vi "DAQ_OPC UA.vi"() -> (0 "Error Out":errorcluster)   [LabVIEW 2017]
uses:
  <vilib>/dex/Flush And Wait Empty Condition.ctl
  <vilib>/Platform/TimedLoop/XDataNode/timing_clust.ctl
  <vilib>/Platform/TimedLoop/XDataNode/nitl_modes.ctl
  <vilib>/Platform/TimedLoop/XDataNode/wakeup.ctl
  <vilib>/DAQmx/read.llb/DAQmx Read (Analog 1D DBL NChan 1Samp).vi
  <vilib>/DAQmx/miscellaneous.llb/DAQmx Fill In Error Info.vi
  <vilib>/Platform/TimedLoop/XDataNode/XDataNode.xnode
  <vilib>/Platform/TimedLoop/XDataNode/XDNodeRunTimeDep.lvlib
  <resource>/objmgr/ni.dex.rc
panel:
  out "Producer Loop Time":i64
  out "Consumer Loop Time":u32
  out "Time":dbl
  out "Available Elements for Writing":i32
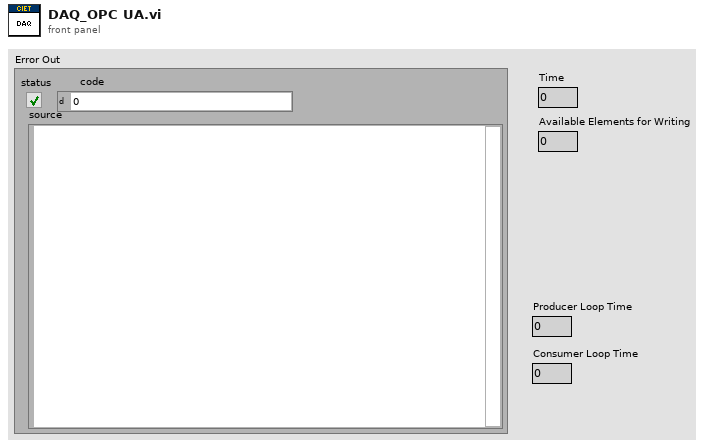
[diagram p1: front panel]
types:
  T1 = typedef "Flush And Wait Empty Condition.ctl" = u8
  T2 = typedef "XDNodeRunTimeDep.lvlib/timing_clust.ctl" = cluster{"Expected End [f-1]":u64, "Actual End [f-1]":u64, "Finished Late? [f-1]":bool, "Expected End [i-1]":u64, "Actual End [i-1]":u64, "Finished Late? [i-1]":bool, "Expected Start [i]":u64, "Actual Start [i]":u64, "Expected Start [f]":u64, "Actual Start [f]":u64, "Source Name":string, "Structure Name":string, "Period":i64, "Deadline":i64, "Offset":i64, "Start":i64, "Priority":i32, "Timeout":i32, "Mode":T3, "Wakeup Reason":T4, "Error":errorcluster, "Source Type":string, "Secondary Source Type":string, "Global End Time":u64, "Global Start Time":u64, "Frame Duration":u64, "Iteration Duration":u64, "Assigned CPU":i32, "I/O Scan Engine Mode":u32}
  T3 = typedef "XDNodeRunTimeDep.lvlib/nitl_modes.ctl" = enum32{"No Change", "Process missed periods, maintain original phase", "Discard missed periods, maintain original phase", "Process missed periods, ignore original phase", "Discard missed periods, ignore original phase"}
  T4 = typedef "XDNodeRunTimeDep.lvlib/wakeup.ctl" = enum32{"Normal", "Aborted", "Asynchronous wakeup", "Timing source error", "Timed loop error", "Timeout"}
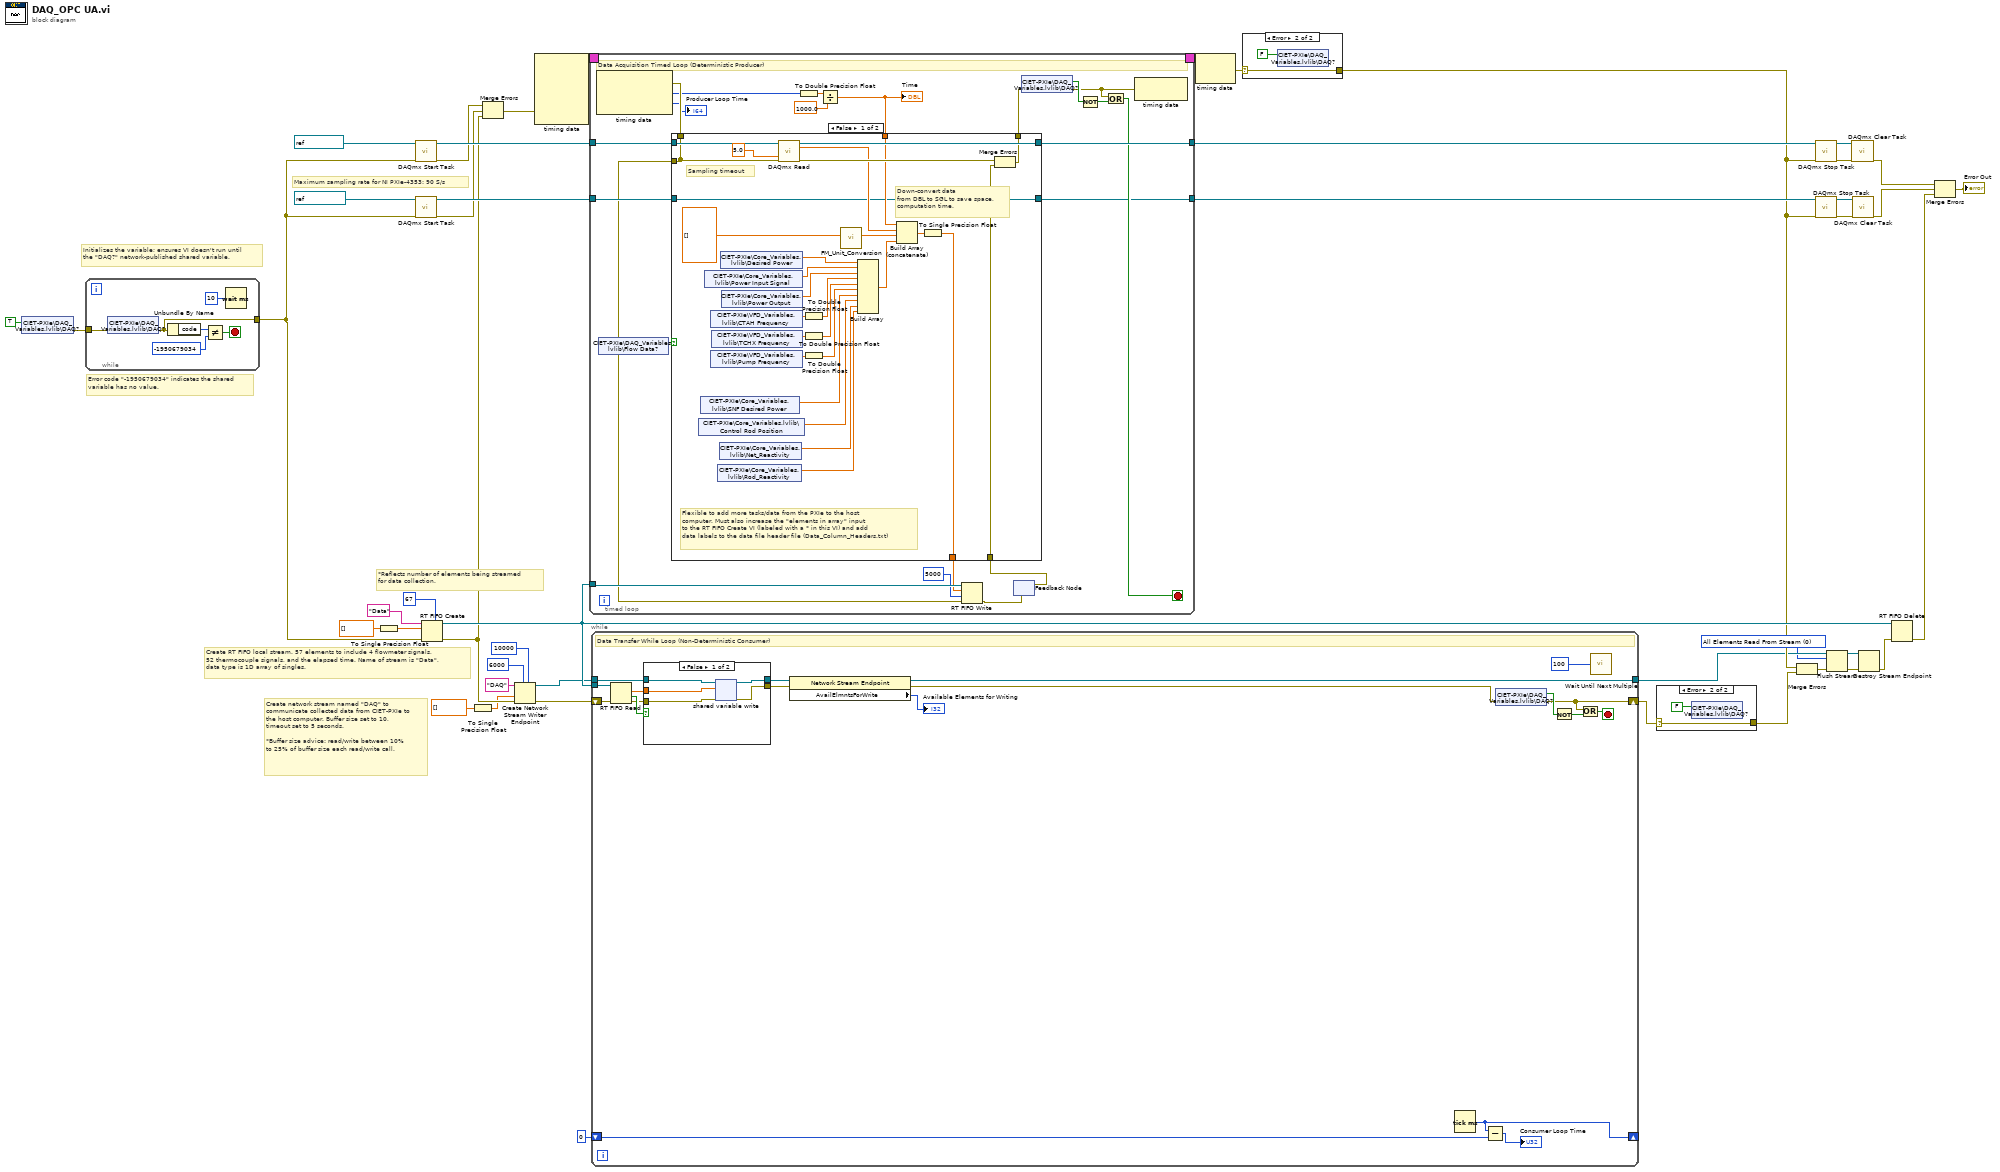
[diagram p0: block diagram]
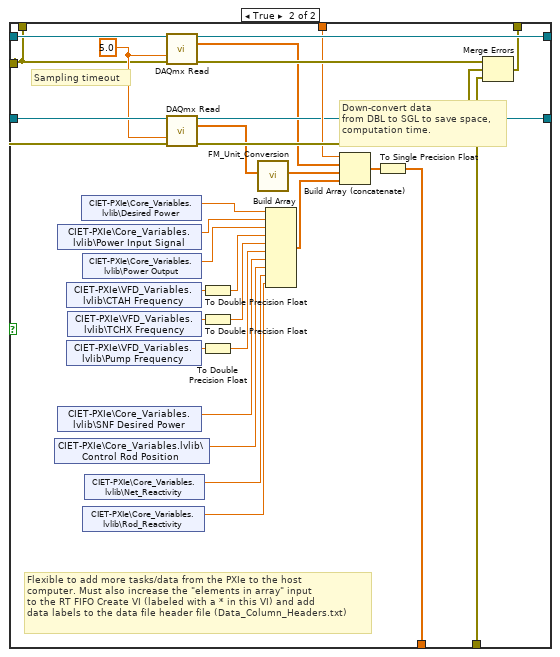
[diagram p5: hidden frame]
diagram:
  w2 = T1 0 items=["All Elements Read From Stream", "All Elements Available for Reading"] ("wait condition")
  # "*Reflects number of elements being streamed\nfor data collection."
  # "Create RT FIFO local stream. 57 elements to include 4 flowmeter signals,\n52 thermocouple signals, and the elapsed time. Name of stream is \"Data\",\ndata type is 1D array of singles."
  # "Create network stream named \"DAQ\" to communicate collected data from CIET-PXIe to the host computer. Buffer size set to 10, timeout set to 5 seconds. \n\n*Buffer size advice: read/write between 10%\nto 25% of buffer size each read/write call."
  # "Maximum sampling rate for NI PXIe-4353: 90 S/s"
  # "Initializes the variable; ensures VI doesn't run until\nthe \"DAQ?\" network-published shared variable."
  # "Error code \"-1950679034\" indicates the shared\nvariable has no value."
  n1 = shared-variable "CIET-PXIe\\DAQ_Variables.lvlib\\DAQ?"(TRUE ("Active?")) -> (error out=w22:errorcluster)  [unwired: 1 in]
  n2 = while {
    tunnel: w22 -> [w51]
    tunnel: [w50] -> w21
    stop <- w47 stop-if-true
    n3 = shared-variable "CIET-PXIe\\DAQ_Variables.lvlib\\DAQ?"(error in=w51) -> (error out=w50:errorcluster)  [unwired: 1 out]
    n4 = Unbundle By Name(w50) -> ("code"=w49:i32)
    n5 = Not Equal?(x=w49, y=-1950679034) -> (x != y?=w47:bool)
    n6 = Wait (ms)(milliseconds to wait=u32 10) -> ()  [unwired: 1 out]
  }
  n7 = To Single Precision Float(number=dbl[] []) -> (single precision float=w32:sgl[])
  n8 = call <vilib>:"DAQmx Start Task.vi"("task/channels in"=refnum<k21> "CIET-TC", "error in"=w21) -> ("task out"=w42:refnum<k21>, "error out"=w26:errorcluster)  [unwired: 12 in]
  n9 = call <vilib>:"DAQmx Start Task.vi"("task/channels in"=refnum<k21> "CIET-FM", "error in"=w21) -> ("task out"=w41:refnum<k21>, "error out"=w27:errorcluster)  [unwired: 12 in]
  n10 = RT FIFO Create(0:"Data" ("name (unnamed)"), 1:w32, 3:w21, 6:u32 67 ("elements in array (1)")) -> (8:w25:refnum<k33>, 11:w17:errorcluster)  [unwired: 4 in, 1 out]
  n11 = To Single Precision Float(number=dbl[] []) -> (single precision float=w7:sgl[])
  n12 = Merge Errors(w26, w27, w17) -> (w28:errorcluster)
  n13 = Create Network Stream Writer Endpoint(5:10000 ("timeout in ms (-1)"), 7:6000 ("writer buffer size"), 8:w17, 9:w7, 11:"DAQ" ("writer name")) -> (0:w18:errorcluster, 3:w16:refnum<k21>)  [unwired: 2 in]
  n14 = node-c288(w28) -> (w46:T2)  [unwired: 4 in]
  n15 = timed-loop {
    timing: w46 -> [_]
    timing-out: [_] -> w45
    tunnel: w25 -> [w71]
    tunnel: w42 -> [w74]
    tunnel: [w72] -> w36
    tunnel: w41 -> [w73]
    tunnel: [w59] -> w35
    stop <- w66 stop-if-true
    # "Data Acquisition Timed Loop (Deterministic Producer)"
    n16 = node-c288() -> (w69:errorcluster, w60:i64, →"Producer Loop Time":i64)  [unwired: 1 in]
    n17 = shared-variable "CIET-PXIe\\DAQ_Variables.lvlib\\Flow Data?"() -> (w54:bool)  [unwired: 1 in, 1 out]
    n18 = To Double Precision Float(number=w60) -> (double precision float=w63:dbl)
    n19 = Divide(x=w63, y=1000.0) -> (x/y=w62:dbl)
    "Time" <- w62
    n20 = feedback #1() -> (w55:errorcluster)  [unwired: 1 in]
    n21 = case shown="False" w54 {
      tunnel: w74 -> [w102 w132]
      tunnel: w73 -> [w82 w131]
      tunnel: [w100 w129] -> w72
      tunnel: [w98 w127] -> w57
      tunnel: w69 -> [w79 w107]
      tunnel: w55 -> [w80 w124]
      tunnel: [w96 w123] -> w65
      tunnel: w62 -> [w95 w122]
      tunnel: [w82 w121] -> w59
      tunnel: [w79 w107] -> w53
      frame False {
        # "Flexible to add more tasks/data from the PXIe to the host \ncomputer. Must also increase the \"elements in array\" input \nto the RT FIFO Create VI (labeled with a * in this VI) and add\ndata labels to the data file header file (Data_Column_Headers.txt)"
        # "Down-convert data\nfrom DBL to SGL to save space,\ncomputation time."
        # "Sampling timeout"
        n22 = shared-variable "CIET-PXIe\\Core_Variables.lvlib\\Control Rod Position"() -> (w77:dbl)  [unwired: 1 in, 1 out]
        n23 = shared-variable "CIET-PXIe\\Core_Variables.lvlib\\SNF Desired Power"() -> (w78:dbl)  [unwired: 1 in, 1 out]
        n24 = shared-variable "CIET-PXIe\\Core_Variables.lvlib\\Power Input Signal"() -> (w85:dbl)  [unwired: 1 in, 1 out]
        n25 = shared-variable "CIET-PXIe\\VFD_Variables.lvlib\\CTAH Frequency"() -> (w87:sgl)  [unwired: 1 in, 1 out]
        n26 = shared-variable "CIET-PXIe\\VFD_Variables.lvlib\\Pump Frequency"() -> (w89:sgl)  [unwired: 1 in, 1 out]
        n27 = shared-variable "CIET-PXIe\\VFD_Variables.lvlib\\TCHX Frequency"() -> (w88:sgl)  [unwired: 1 in, 1 out]
        n28 = shared-variable "CIET-PXIe\\Core_Variables.lvlib\\Rod_Reactivity"() -> (w75:dbl)  [unwired: 1 in, 1 out]
        n29 = shared-variable "CIET-PXIe\\Core_Variables.lvlib\\Net_Reactivity"() -> (w76:dbl)  [unwired: 1 in, 1 out]
        n30 = shared-variable "CIET-PXIe\\Core_Variables.lvlib\\Desired Power"() -> (w84:dbl)  [unwired: 1 in, 1 out]
        n31 = shared-variable "CIET-PXIe\\Core_Variables.lvlib\\Power Output"() -> (w86:dbl)  [unwired: 1 in, 1 out]
        n32 = call-poly <vilib>:"DAQmx Read.vi"("task/channels in"=w102, "timeout"=5.0, "error in"=w79) -> ("task out"=w100:refnum<k21>, "data"=w94:dbl[], "error out"=w97:errorcluster)  [unwired: 10 in]
        n33 = To Double Precision Float(number=w87) -> (double precision float=w90:dbl)
        n34 = To Double Precision Float(number=w88) -> (double precision float=w91:dbl)
        n35 = To Double Precision Float(number=w89) -> (double precision float=w92:dbl)
        n36 = call "FM_Unit_Conversion.vi"("Input Array [A]"=dbl[] []) -> ("Output Array [kg/h]"=w93:dbl[])  [unwired: 10 in]
        n37 = Build Array(w84, w85, w86, w90, w91, w92, w78, w77, w76, w75) -> (w83:dbl[])
        n38 = Build Array (concatenate)(w95, w94, w93, w83) -> (w99:dbl[])
        n39 = To Single Precision Float(number=w99) -> (single precision float=w98:sgl[])
        n40 = Merge Errors(w97, w80) -> (w96:errorcluster)
      }
      frame True {
        w130 = 5.0 ("timeout")
        # "Flexible to add more tasks/data from the PXIe to the host \ncomputer. Must also increase the \"elements in array\" input \nto the RT FIFO Create VI (labeled with a * in this VI) and add\ndata labels to the data file header file (Data_Column_Headers.txt)"
        # "Down-convert data\nfrom DBL to SGL to save space,\ncomputation time."
        # "Sampling timeout"
        n41 = shared-variable "CIET-PXIe\\Core_Variables.lvlib\\Control Rod Position"() -> (w105:dbl)  [unwired: 1 in, 1 out]
        n42 = shared-variable "CIET-PXIe\\Core_Variables.lvlib\\Power Input Signal"() -> (w110:dbl)  [unwired: 1 in, 1 out]
        n43 = shared-variable "CIET-PXIe\\Core_Variables.lvlib\\SNF Desired Power"() -> (w106:dbl)  [unwired: 1 in, 1 out]
        n44 = shared-variable "CIET-PXIe\\VFD_Variables.lvlib\\CTAH Frequency"() -> (w112:sgl)  [unwired: 1 in, 1 out]
        n45 = shared-variable "CIET-PXIe\\VFD_Variables.lvlib\\Pump Frequency"() -> (w114:sgl)  [unwired: 1 in, 1 out]
        n46 = shared-variable "CIET-PXIe\\VFD_Variables.lvlib\\TCHX Frequency"() -> (w113:sgl)  [unwired: 1 in, 1 out]
        n47 = shared-variable "CIET-PXIe\\Core_Variables.lvlib\\Desired Power"() -> (w109:dbl)  [unwired: 1 in, 1 out]
        n48 = shared-variable "CIET-PXIe\\Core_Variables.lvlib\\Power Output"() -> (w111:dbl)  [unwired: 1 in, 1 out]
        n49 = shared-variable "CIET-PXIe\\Core_Variables.lvlib\\Rod_Reactivity"() -> (w103:dbl)  [unwired: 1 in, 1 out]
        n50 = shared-variable "CIET-PXIe\\Core_Variables.lvlib\\Net_Reactivity"() -> (w104:dbl)  [unwired: 1 in, 1 out]
        n51 = call-poly <vilib>:"DAQmx Read.vi"("task/channels in"=w132, "timeout"=w130, "error in"=w107) -> ("task out"=w129:refnum<k21>, "data"=w120:dbl[], "error out"=w125:errorcluster)  [unwired: 10 in]
        n52 = call-poly <vilib>:"DAQmx Read.vi"("task/channels in"=w131, "timeout"=w130, "error in"=w107) -> ("task out"=w121:refnum<k21>, "data"=w118:dbl[], "error out"=w126:errorcluster)  [unwired: 10 in]
        n53 = To Double Precision Float(number=w112) -> (double precision float=w115:dbl)
        n54 = To Double Precision Float(number=w113) -> (double precision float=w116:dbl)
        n55 = To Double Precision Float(number=w114) -> (double precision float=w117:dbl)
        n56 = call "FM_Unit_Conversion.vi"("Input Array [A]"=w118) -> ("Output Array [kg/h]"=w119:dbl[])  [unwired: 10 in]
        n57 = Build Array(w109, w110, w111, w115, w116, w117, w106, w105, w104, w103) -> (w108:dbl[])
        n58 = Build Array (concatenate)(w122, w120, w119, w108) -> (w128:dbl[])
        n59 = To Single Precision Float(number=w128) -> (single precision float=w127:sgl[])
        n60 = Merge Errors(w125, w126, w124) -> (w123:errorcluster)
      }
    }
    n61 = RT FIFO Write(0:w71, 1:w57, 2:5000 ("timeout in ms (0)"), 3:w53) -> (11:w56:errorcluster)  [unwired: 1 in, 3 out]
    n62 = feedback-in #1(w56) -> ()
    n63 = shared-variable "CIET-PXIe\\DAQ_Variables.lvlib\\DAQ?"(error in=w65) -> (w68:bool, error out=w64:errorcluster)
    n64 = Not(x=w68) -> (.not. x?=w67:bool)
    n65 = Or(x=w64, y=w67) -> (x .or. y?=w66:bool)
    n66 = node-c288(w64) -> ()  [unwired: 1 out]
  }
  n67 = while {
    tunnel: w25 -> [w158]
    shift-right: [w147] -> w19
    shift-left: w18 -> [w157]
    tunnel: w16 -> [w149]
    tunnel: [w144] -> w9
    shift-right: [w142] -> _
    shift-left: u32 0 ("millisecond timer value") -> [w141]
    stop <- w150 stop-if-true
    # "Data Transfer While Loop (Non-Deterministic Consumer)"
    n68 = RT FIFO Read(0:w158, 3:w157) -> (9:w154:sgl[], 10:w155:bool, 11:w153:errorcluster)  [unwired: 2 in, 2 out]
    n69 = case shown="False" w155 {
      tunnel: w154 -> [w159 _]
      tunnel: w153 -> [w163 w165]
      tunnel: [w162 w165] -> w146
      tunnel: w149 -> [w161 w164]
      tunnel: [w160 w164] -> w145
      frame False {
        n70 = shared-variable-write(w161, w163, w159) -> (w160:refnum<k21>, w162:errorcluster)  [unwired: 1 in, 1 out]
      }
      frame True {
      }
    }
    n71 = property class="Network Stream Endpoint"(reference=w145, error in=w146) -> (reference out=w144:refnum<k21>, error out=w143:errorcluster, "AvailElmntsForWrite"=→"Available Elements for Writing":i32)
    n72 = Tick Count (ms)() -> (millisecond timer value=w142:u32)
    n73 = Subtract(x=w142, y=w141) -> (x-y=→"Consumer Loop Time":u32)
    n74 = shared-variable "CIET-PXIe\\DAQ_Variables.lvlib\\DAQ?"(error in=w143) -> (w152:bool, error out=w147:errorcluster)
    n75 = Not(x=w152) -> (.not. x?=w151:bool)
    n76 = Or(x=w147, y=w151) -> (x .or. y?=w150:bool)
    n77 = call "Wait Until Next Multiple"("Count(mSec)"=u32 100) -> ()  [unwired: 1 out]
  }
  n78 = node-c288(w45) -> (w20:errorcluster)
  n79 = case shown="Error" w20 {
    selector: w20 -> [w166 w167]
    tunnel: [w166 w167] -> w15
    frame No Error {
    }
    frame Error {
      n80 = shared-variable "CIET-PXIe\\DAQ_Variables.lvlib\\DAQ?"(FALSE ("DAQ?")) -> ()  [unwired: 1 in, 1 out]
    }
  }
  n81 = case shown="Error" w19 {
    selector: w19 -> [w169 w170]
    tunnel: [w169 w170] -> w14
    frame No Error {
    }
    frame Error {
      n82 = shared-variable "CIET-PXIe\\DAQ_Variables.lvlib\\DAQ?"(FALSE ("DAQ?")) -> ()  [unwired: 1 in, 1 out]
    }
  }
  n83 = Merge Errors(w15, w14) -> (w11:errorcluster)
  n84 = call <vilib>:"DAQmx Stop Task.vi"("task/channels in"=w36, "error in"=w15) -> ("task out"=w39:refnum<k21>, "error out"=w40:errorcluster)  [unwired: 12 in]
  n85 = call <vilib>:"DAQmx Stop Task.vi"("task/channels in"=w35, "error in"=w15) -> ("task out"=w37:refnum<k21>, "error out"=w38:errorcluster)  [unwired: 12 in]
  n86 = Flush Stream(8:w11, 10:w2, 11:w9) -> (0:w13:errorcluster, 3:w12:refnum<k21>)  [unwired: 1 in, 1 out]
  n87 = call <vilib>:"DAQmx Clear Task.vi"("task in"=w39, "error in"=w40) -> ("error out"=w34:errorcluster)  [unwired: 13 in]
  n88 = call <vilib>:"DAQmx Clear Task.vi"("task in"=w37, "error in"=w38) -> ("error out"=w33:errorcluster)  [unwired: 13 in]
  n89 = Destroy Stream Endpoint(8:w13, 11:w12) -> (0:w10:errorcluster)
  n90 = RT FIFO Delete(0:w25, 3:w10) -> (11:w4:errorcluster)  [unwired: 1 in]
  n91 = Merge Errors(w34, w33, w4) -> (→"Error Out":errorcluster)
